vi "LinearFilter_LP_BW2_Execute.vi"(8 "SamplePeriod":dbl=0.02 format="%13.5f", 9 "TimeConstant":dbl=0.02 format="%13.5f", 10 "Enable":bool=TRUE, 11 "Input":dbl format="%13.5p") -> (1 "Output":dbl format="%13.5p")   [LabVIEW 2019, in "Trajectory_Library.lvlib"]
doc: "This is a LabVIEW \"convience\" function that combines the various subVI for a linear filter into a single subVI. This subVI creates and executes the linear filter. The filter can be dynamically enabled and disabled. When the filter is disabled, the input is transfered directly to the output. Bumpless transfer is provided when enabling the filter. Bumpless transfer is NOT provided when disabling the filter. The output value jumps directly to the current input value. The filter type and filter constants can also be changed dynamically. When the filter contstants are changed, the output may jump to the current input value when the internal buffers are reset to the current input value.\n\nInputs:\n - FilterType - An enumerated value used to select the type of filter to be cofigured. The possible values are:\n - Moving Average - Specify the \"sample\" input.\n - Low pass 1st order Butterworth filter\n - Low pass 2nd order Butterworth filter\n - High pass 1st order Butterworth filter\n - High pass 2nd order Butterworth filter\n - Input - Input value to be filtered (Required) \n - Enable - Boolean indicating filtering should be performed (Default = True)\n - TimeConstant - Filtering time constant seconds. Used for all types except Moving \n Average (Default = 0.020) \n - SamplePeriod - Execution period seconds. Used for all types except Moving Average. \n (Default = 0.020)\n - Samples - Number of samples for the moving average filter. (Default = 3)\n\nOutputs:\n - OutLinearFilter - Current value of the LinearFilter data structure.\n - Output - Current output value."
uses:
  Trajectory_Library.lvlib
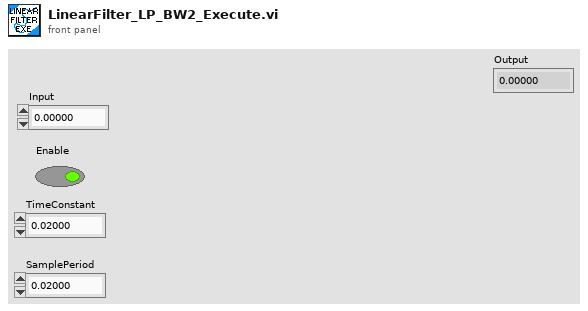
[diagram p1: front panel]
types:
  T1 = typedef "Trajectory_Library.lvlib/LINEAR_FILTER.ctl" = cluster{"InputGains":dbl[], "OutputGains":dbl[], "Inputs":dbl[], "Outputs":dbl[], "InGainCount":i32, "OutGainCount":i32}
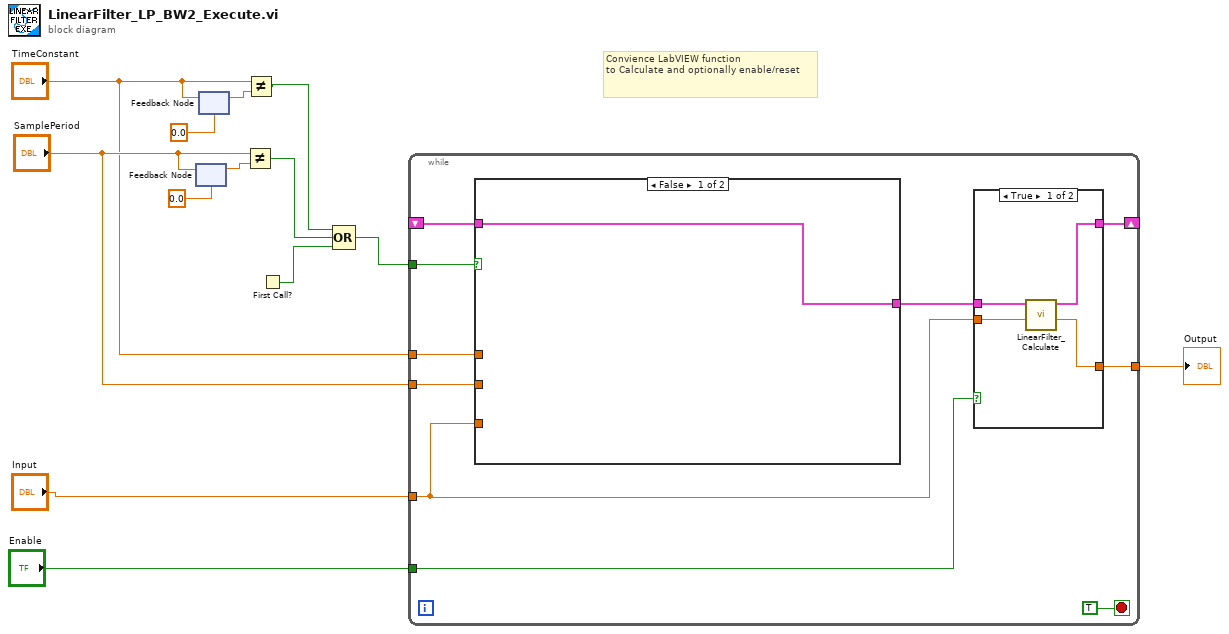
[diagram p0: block diagram]
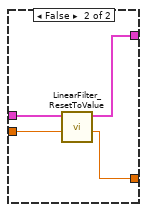
[diagram p2: hidden frame]
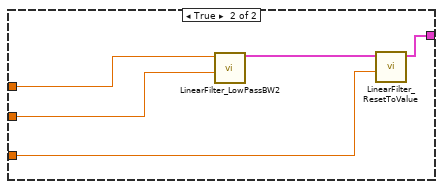
[diagram p3: hidden frame]
diagram:
  # "Convience LabVIEW function\nto Calculate and optionally enable/reset"
  n1 = feedback #1(0.0 ("SamplePeriod")) -> (w4:dbl)
  n2 = feedback-in #1("SamplePeriod") -> ()
  n3 = feedback #2(0.0 ("TimeConstant")) -> (w5:dbl)
  n4 = feedback-in #2("TimeConstant") -> ()
  n5 = Not Equal?(x="SamplePeriod", y=w4) -> (x != y?=w9:bool)
  n6 = Not Equal?(x="TimeConstant", y=w5) -> (x != y?=w10:bool)
  n7 = First Call?() -> (First Call?: T/F=w8:bool)
  n8 = Compound Arithmetic op=OR(w10, w9, w8) -> (w3:bool)
  n9 = while {
    tunnel: "Enable" -> [w23]
    tunnel: "SamplePeriod" -> [w19]
    tunnel: "TimeConstant" -> [w18]
    tunnel: w3 -> [w16]
    tunnel: "Input" -> [w21]
    tunnel: [w22] -> w12
    shift-right: [w17] -> _
    shift-left: _ -> [w14]
    stop <- TRUE stop-if-true
    n10 = case shown="False" w16 {
      tunnel: w19 -> [_ w35]
      tunnel: w18 -> [_ w34]
      tunnel: w21 -> [_ w33]
      tunnel: [w31 w32] -> w20
      tunnel: w14 -> [w31 _]
      frame False {
      }
      frame True {
        n11 = call "LinearFilter_LowPassBW2.vi"("SamplePeriod"=w35, "TimeConstant"=w34) -> ("LINEAR_FILTER"=w36:T1)  [unwired: 9 in]
        n12 = call "LinearFilter_ResetToValue.vi"("InputValue"=w33, "In LINEAR_FILTER"=w36) -> ("Out LINEAR_FILTER"=w32:T1)  [unwired: 9 in]
      }
    }
    n13 = case shown="True" w23 {
      tunnel: w20 -> [w27 w30]
      tunnel: [w26 w29] -> w17
      tunnel: w21 -> [w25 w28]
      tunnel: [w24 w28] -> w22
      frame True {
        n14 = call "LinearFilter_Calculate.vi"("Input"=w25, "In LINEAR_FILTER"=w27) -> ("Output"=w24:dbl, "Out LINEAR_FILTER"=w26:T1)  [unwired: 8 in]
      }
      frame False {
        n15 = call "LinearFilter_ResetToValue.vi"("InputValue"=w28, "In LINEAR_FILTER"=w30) -> ("Out LINEAR_FILTER"=w29:T1)  [unwired: 9 in]
      }
    }
  }
  "Output" <- w12
